vi "Configure Sweep.vi"(6 "Interval (1.0 ms)":dbl=1.0, 8 "error in (no error)":errorcluster, 9 "Sweep Points (1)":u32=1, 10 "Channel (1: Channel 1)":u16(ring)=1 items=["Channel 1"=1, "Channel 2"=2, "Channel 3"=3], 11 "VISA resource name":refnum<visa-resource-name>) -> (0 "error out":errorcluster, 3 "VISA resource name out":refnum<visa-resource-name>)   [LabVIEW 2010, in "Agilent U2722.lvlib"]
doc: "Configures how the instrument measures multiple points."
uses:
  Agilent U2722.lvlib
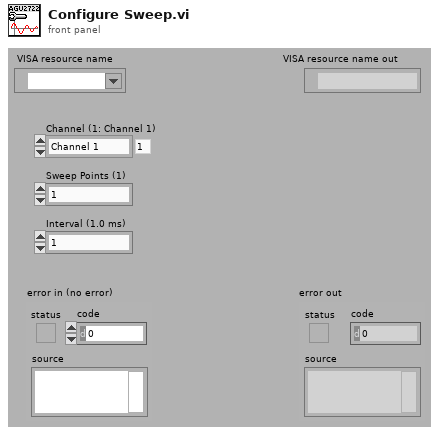
[diagram p1: front panel]
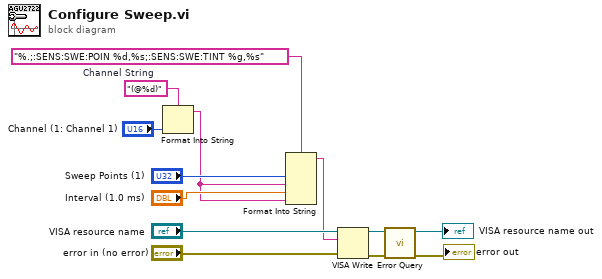
[diagram p0: block diagram]
diagram:
  w8 = "(@%d)"  # Channel String
  n1 = Format Into String(format string=w8, "Channel (1: Channel 1)") -> (resulting string=w2:string)  [unwired: 2 in, 1 out]
  n2 = Format Into String(format string="%.;:SENS:SWE:POIN %d,%s;:SENS:SWE:TINT %g,%s", "Sweep Points (1)", w2, "Interval (1.0 ms)", w2) -> (resulting string=w1:string)  [unwired: 2 in, 1 out]
  n3 = VISA Write(VISA resource name="VISA resource name", write buffer=w1, error in (no error)="error in (no error)") -> (VISA resource name out=w11:refnum<visa-resource-name>, error out=w10:errorcluster)  [unwired: 1 out]
  n4 = call "Error Query.vi"("error in (no error)"=w10, "VISA resource name"=w11) -> ("error out"=→"error out":errorcluster, "VISA resource name out"=→"VISA resource name out":refnum<visa-resource-name>)  [unwired: 6 in, 2 out]
